vi "PCO_OpenCamera.vi"(3 "error in (no error)":errorcluster, 4 "Handle (0 for new)":u64) -> (0 "error out":errorcluster, 1 "Handle Out":u64, 2 "return type":u32 format="%.0x")   [LabVIEW 2011]
uses:
  SC2_Cam64.dll
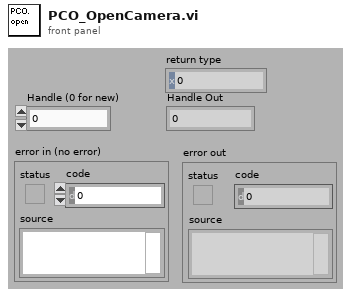
[diagram p1: front panel]
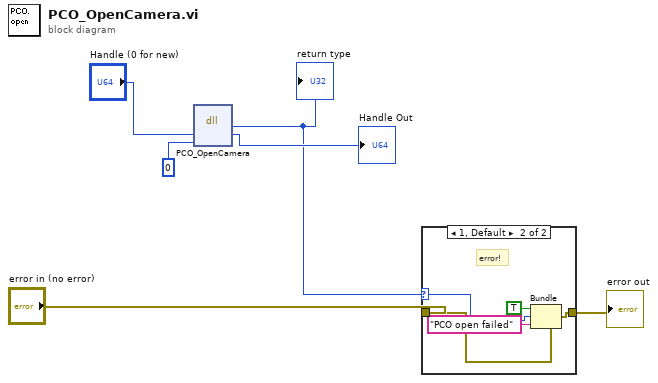
[diagram p0: block diagram]
diagram:
  n1 = dll-call lib="SC2_Cam*.*" fn="PCO_OpenCamera"("Handle"="Handle (0 for new)", "dummy"=i16 0) -> ("return type"=w3:u32, "Handle"=→"Handle Out":u64)  [unwired: 4 in, 2 out]
  "return type" <- w3
  n2 = case shown="1, Default" w3 {
    selector: w3 -> [_ w9]
    tunnel: "error in (no error)" -> [w7 w11]
    tunnel: [w7 w12] -> w1
    frame 0 {
    }
    frame 1, Default {
      # "error!"
      n3 = Bundle(cluster=w11, "status"=TRUE, "code"=w9, "source"="PCO open failed") -> (w12:errorcluster)
    }
  }
  "error out" <- w1
